vi "Get Default Project Path.vi"(11 "error in":errorcluster) -> (4 "Project Path":path, 15 "error out":errorcluster)   [LabVIEW 2021, in "Path Functions.lvlib"]
uses:
  Path Functions.lvlib
  <vilib>/Utility/sysdir.llb/System Directory Type.ctl
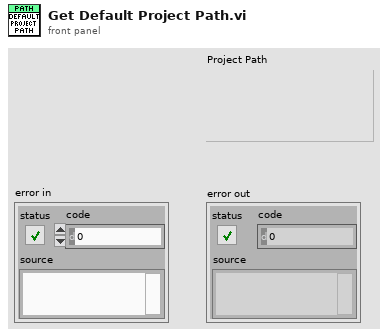
[diagram p1: front panel]
types:
  T1 = typedef "System Directory Type.ctl" = i32
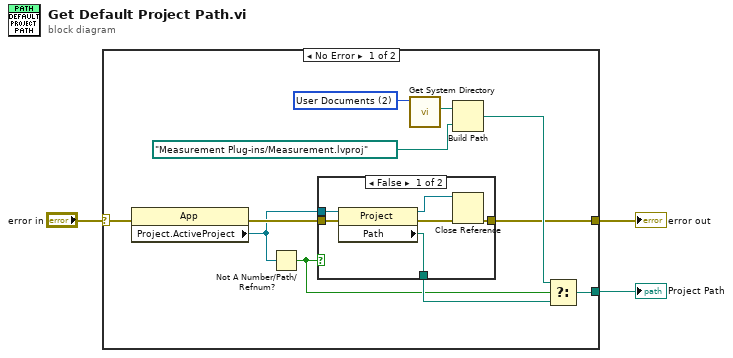
[diagram p0: block diagram]
diagram:
  n1 = case shown="No Error" "error in" {
    selector: "error in" -> [w13 w22]
    tunnel: [w7 w22] -> w2
    tunnel: [w6 _] -> w1
    frame No Error {
      w10 = T1 2 items=["User Home"=0, "User Desktop"=1, "User Documents"=2, "User Application Data"=3, "User Preferences"=4, "User Temporary"=5, "Public Documents"=6, "Public Application Data"=7, "Public Preferences"=8, "Public Cache"=13, "System Core Libraries"=9, "System Installed Libraries"=10, "Application Files"=11, "Boot Volume Root"=12] ("system directory type")
      n2 = property class="App"(error in=w13) -> (error out=w14:errorcluster, "Project.ActiveProject"=w5:refnum<vi>)  [unwired: 1 in, 1 out]
      n3 = Not A Number/Path/Refnum?(number/path/refnum=w5) -> (NaN/Path/Refnum?=w4:bool)
      n4 = case shown="False" w4 {
        tunnel: w14 -> [w18 w21]
        tunnel: [w17 _] -> w8
        tunnel: [w16 w21] -> w7
        tunnel: w5 -> [w15 _]
        frame False {
          n5 = property class="Project"(reference=w15, error in=w18) -> (reference out=w20:refnum<vi>, error out=w19:errorcluster, "Path"=w17:path)
          n6 = Close Reference(reference=w20, error in (no error)=w19) -> (error out=w16:errorcluster)
        }
        frame True {
        }
      }
      n7 = call <vilib>:"Get System Directory.vi"("system directory type"=w10) -> ("system directory"=w11:path)  [unwired: 10 in]
      n8 = Build Path(base path=w11, name or relative path=path "Measurement Plug-ins/Measurement.lvproj") -> (appended path=w9:path)
      n9 = Select(t=w9, s=w4, f=w8) -> (s? t:f=w6:path)
    }
    frame Error {
    }
  }
  "error out" <- w2
  "Project Path" <- w1
